vi "Set Domain.vi"(8 "error in (no error)":errorcluster, 10 "domain":variant, 11 "Domain_Steady_2D_Rect in":refnum<class "NI_Domain_Steady_2D_Rect.lvclass">) -> (0 "error out":errorcluster, 3 "Domain_Steady_2D_Rect out":refnum<class "NI_Domain_Steady_2D_Rect.lvclass">)   [LabVIEW 2020, in "NI_PDE.lvlib" / "NI_Domain_Steady_2D_Rect.lvclass"]
uses:
  <vilib>/gmath/pde.llb/DomainClass/Domain_Steady_2D_Rect/NI_Domain_Steady_2D_Rect.lvclass
  <vilib>/gmath/pde.llb/DomainClass/Domain_Steady_2D_Rect/Domain Data.ctl
  <vilib>/gmath/pde.llb/DomainClass/Domain_Steady_2D_Rect/NI_Domain_Steady_2D_Rect.lvclass/NI_Domain_Steady_2D_Rect.ctl
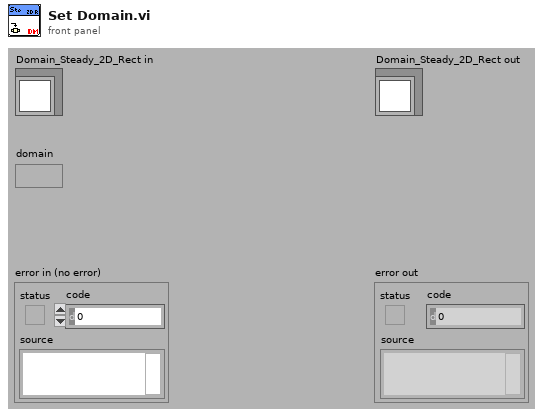
[diagram p1: front panel]
types:
  T1 = typedef "NI_PDE.lvlib/NI_Domain_Steady_2D_Rect.lvclass/Domain Data.ctl" = cluster{"X":cluster{"start x":dbl, "end x":dbl, "# of x-points":i32}, "Y":cluster{"start y":dbl, "end y":dbl, "# of y-points":i32}}
  T2 = cluster{"start x":dbl, "end x":dbl, "# of x-points":i32}
  T3 = cluster{"start y":dbl, "end y":dbl, "# of y-points":i32}
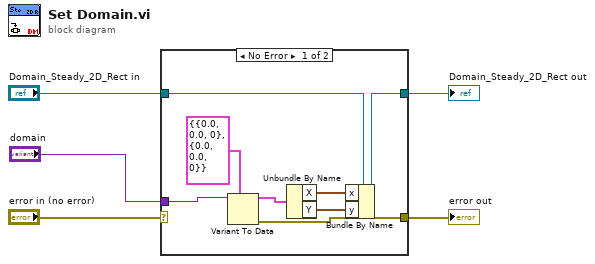
[diagram p0: block diagram]
diagram:
  n1 = case shown="No Error" "error in (no error)" {
    selector: "error in (no error)" -> [_ w15]
    tunnel: "Domain_Steady_2D_Rect in" -> [w10 w14]
    tunnel: [w9 w14] -> w5
    tunnel: [w8 w15] -> w4
    tunnel: "domain" -> [w13 _]
    frame No Error {
      n2 = Variant To Data(type=T1 {"X"={"start x"=0.0, "end x"=0.0, "# of x-points"=0}, "Y"={"start y"=0.0, "end y"=0.0, "# of y-points"=0}} ("domain data"), Variant=w13) -> (data=w11:T1, error out=w8:errorcluster)  [unwired: 1 in]
      n3 = Unbundle By Name(w11) -> ("X"=w7:T2, "Y"=w6:T3)
      n4 = Bundle By Name(cluster=w10, "x"=w7, "y"=w6) -> (w9:refnum<class "NI_Domain_Steady_2D_Rect.lvclass">)
    }
    frame Error {
    }
  }
  "Domain_Steady_2D_Rect out" <- w5
  "error out" <- w4
